vi "Get System Parameter(Array).vi"(8 "error in (no error)":errorcluster caption="错误输入（无错误）", 10 "propertyName":string="IPENABLED", 11 "path":string="Win32_NetworkAdapterConfiguration") -> (0 "error out":errorcluster caption="错误输出", 3 "Parameters":string[](array[string])=["False", "False", "False", "False", "False", "False", "True", "False", "True", "False", "False", "False"])   [LabVIEW 2013, in "ManagementClass.lvclass"]
uses:
  ManagementClass.lvclass
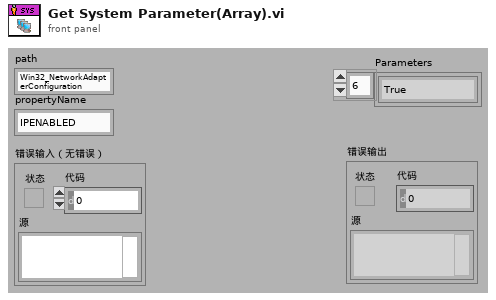
[diagram p1: front panel]
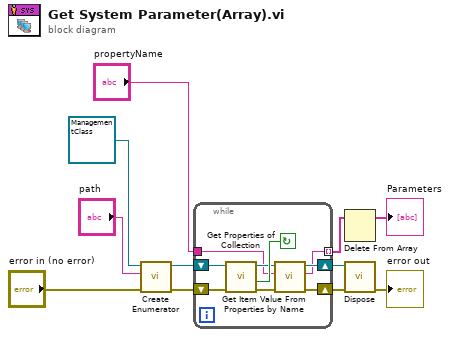
[diagram p0: block diagram]
diagram:
  n1 = call "Create Enumerator.vi"("error in (no error)"="error in (no error)", "path"="path", "ManagementClass 输入"=refnum<class "ManagementClass.lvclass"> refnum) -> ("error out"=w9:errorcluster, "ManagementClass 输出"=w10:refnum<class "ManagementClass.lvclass">)  [unwired: 7 in]
  n2 = while {
    shift-right: [w14] -> w7
    shift-left: w10 -> [w20]
    shift-right: [w15] -> w8
    shift-left: w9 -> [w17]
    tunnel: [w13] -> w2 mode=indexing
    tunnel: "propertyName" -> [w12]
    stop <- w19 continue-if-true
    n3 = call "Get Properties of Collection.vi"("error in (no error)"=w17, "ManagementClass 输入"=w20) -> ("error out"=w16:errorcluster, "非空"=w19:bool, "ManagementClass 输出"=w18:refnum<class "ManagementClass.lvclass">)  [unwired: 7 in]
    n4 = call "Get Item Value From Properties by Name.vi"("error in (no error)"=w16, "PropertyName"=w12, "ManagementClass 输入"=w18) -> ("error out"=w15:errorcluster, "Value"=w13:string, "ManagementClass 输出"=w14:refnum<class "ManagementClass.lvclass">)  [unwired: 6 in]
  }
  n5 = Delete From Array(array=w2) -> (array with subset deleted=→"Parameters":string[])  [unwired: 2 in, 1 out]
  n6 = call "Dispose.vi"("error in (no error)"=w8, "ManagementClass 输入"=w7) -> ("error out"=→"error out":errorcluster)  [unwired: 9 in]
